vi "Fix Saturated Sin.vi"(9 "start index (0)":i32, 11 "Waveform":dbl[](array[numeric])) -> (0 "RMS value":dbl format="%0.2p", 1 "Rising":i32, 2 "1/2 Period":i32, 3 "Falling":i32, 4 "Sat. Ind":u64, 5 "Peak Amplitude":dbl, 6 "Error":dbl format="%0.6f", 7 "Waveform Graph":dbl[][](graph))   [LabVIEW 2017]
uses:
  <vilib>/Analysis/baseanly.llb/Mean (DBL).vi
  <vilib>/measure/madcrms.llb/Basic Averaged DC-RMS for 1 Chan.vi
  <vilib>/measure/NI_MAPro.lvlib
  <vilib>/Analysis/NI_AALPro.lvlib
  <vilib>/Analysis/2dsp.llb/Real FFT.vi
  <vilib>/measure/mamon.llb/Trigger Detection for 1 Channel.vi
  Crabtree-Lab-Panel--master/Crabtree LAB Panel/Lab Panel V2/program files/Global 1.vi
  <vilib>/Analysis/NI_AALBase.lvlib
panel:
  out "Waveform Graph 3":dbl[](graph)
  out "x-y":dbl[](array[numeric])
  out "Waveform Graph 2":dbl[][](graph)
  in  "O/P Sin Scaler":dbl=1.0
  in  "Threshoild level":dbl=5.0 format="%#_13g"
  in  "Scaling":dbl=1.0
  # "e"
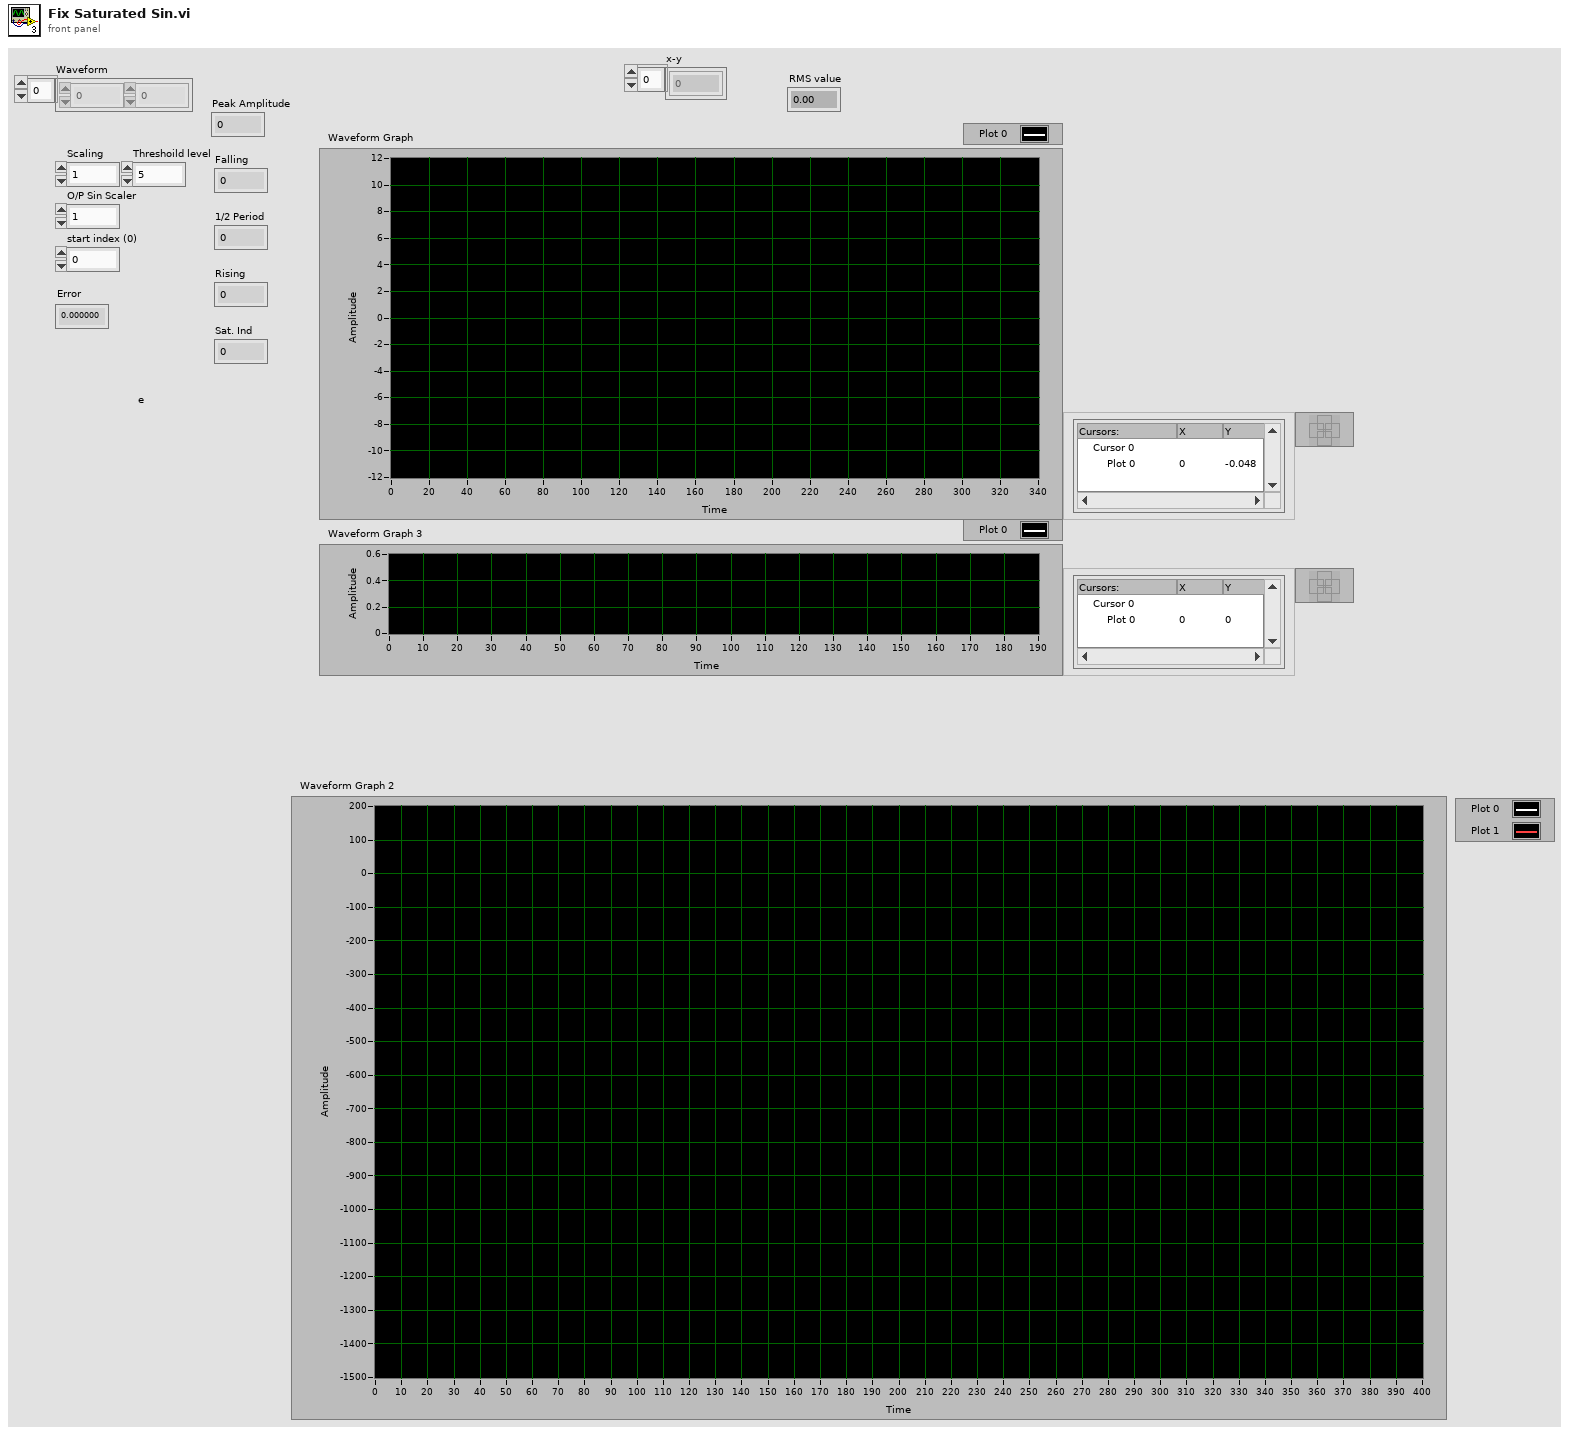
[diagram p1: front panel]
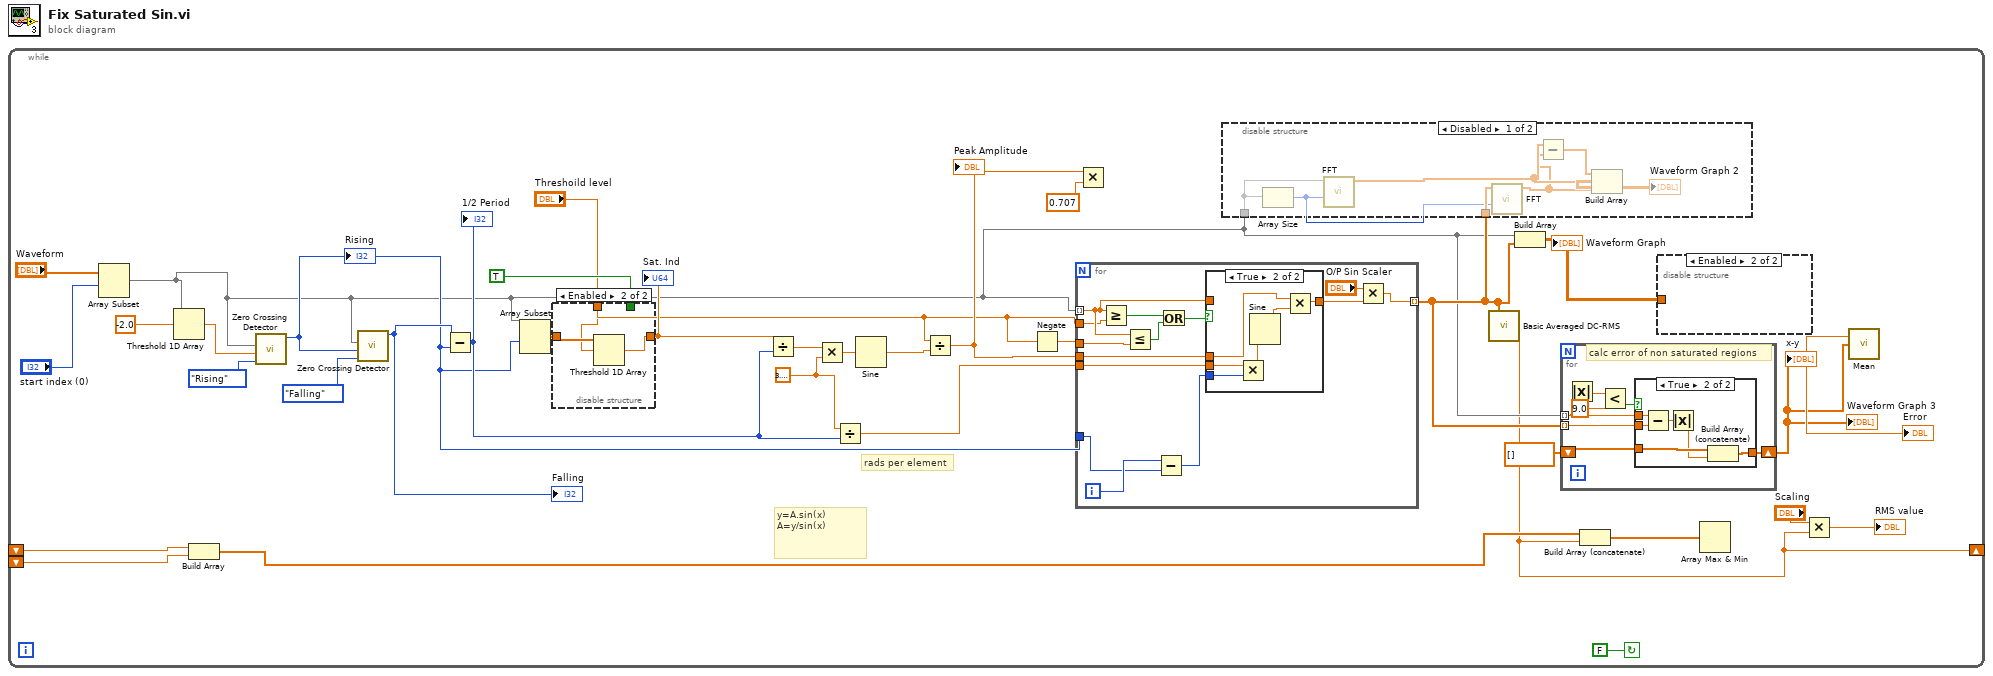
[diagram p0: block diagram]
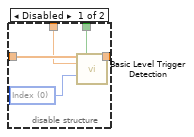
[diagram p3: hidden frame]
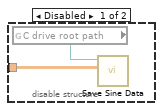
[diagram p4: hidden frame]
diagram:
  n1 = while {
    shift-right: [w2] -> _
    shift-left: _ -> [w16]
    shift-left: _ -> [w17]
    stop <- FALSE continue-if-true
    w25 = 3.141592653589793
    # "y=A.sin(x)\nA=y/sin(x)"
    # "rads per element"
    n2 = Array Subset(array="Waveform", index="start index (0)") -> (w6:dbl[])  [unwired: 1 in]
    n3 = Threshold 1D Array(2:-2.0 ("threshold y"), 3:w6) -> (0:w11:dbl)  [unwired: 1 in]
    n4 = Build Array(w17, w16) -> (w15:dbl[])
    n5 = call "Zero Crossing Detector.vi"("Direction"=enum16{"Rising", "Falling"}."Rising", "offset"=w11, "Y"=w6) -> ("X"=w22:i32)  [unwired: 8 in]
    "Rising" <- w22
    n6 = call "Zero Crossing Detector.vi"("Direction"=enum16{"Rising", "Falling"}."Falling", "offset"=w22, "Y"=w6) -> ("X"=w29:i32)  [unwired: 8 in]
    "Falling" <- w29
    n7 = Subtract(x=w29, y=w22) -> (x-y=w24:i32)
    "1/2 Period" <- w24
    n8 = Array Subset(array=w6, index=w22) -> (w31:dbl[])  [unwired: 1 in]
    n9 = disable-structure shown="Enabled" {
      disable-tunnel: [w54 w55] -> w32
      disable-tunnel: w31 -> [w53 w57]
      disable-tunnel: TRUE ("reset") -> [w51 _]
      disable-tunnel: "Threshoild level" -> [w50 w56]
      frame Disabled {
        w52 = u16 0 items=["Index", "Time"] ("location mode")
        n10 = call-poly <vilib>:"Basic Level Trigger Detection.vi"("signal in"=w53, "reset"=w51, "level"=w50, "location mode"=w52) -> ("trigger location"=w54:dbl)  [unwired: 9 in, 2 out]
      }
      frame Enabled {
        n11 = Threshold 1D Array(2:w56, 3:w57) -> (0:w55:dbl)  [unwired: 1 in]
      }
    }
    "Sat. Ind" <- w32
    n12 = Divide(x=w32, y=w24) -> (x/y=w33:dbl)
    n13 = Multiply(x=w33, y=w25) -> (x*y=w34:dbl)
    n14 = Divide(x=w25, y=w24) -> (x/y=w23:dbl)
    n15 = Sine(x=w34) -> (sin(x)=w35:dbl)
    n16 = Divide(x="Threshoild level", y=w35) -> (x/y=w21:dbl)
    "Peak Amplitude" <- w21
    n17 = Negate(x="Threshoild level") -> (-x=w19:dbl)
    n18 = for {
      tunnel: w6 -> [w73] mode=indexing
      tunnel: "Threshoild level" -> [w72]
      tunnel: w23 -> [w80]
      tunnel: w21 -> [w79]
      tunnel: [w68] -> w10 mode=indexing
      tunnel: w22 -> [w77]
      tunnel: w19 -> [w70]
      i -> [w78]
      n19 = Greater Or Equal?(x=w73, y=w72) -> (x >= y?=w74:bool)
      n20 = Less Or Equal?(x=w73, y=w70) -> (x <= y?=w71:bool)
      n21 = Subtract(x=w78, y=w77) -> (x-y=w76:i32)
      n22 = Or(x=w74, y=w71) -> (x .or. y?=w75:bool)
      n23 = case shown="True" w75 {
        tunnel: [w81 w82] -> w69
        tunnel: w73 -> [w81 _]
        tunnel: w76 -> [_ w87]
        tunnel: w80 -> [_ w86]
        tunnel: w79 -> [_ w83]
        frame False {
        }
        frame True {
          n24 = Multiply(x=w86, y=w87) -> (x*y=w85:dbl)
          n25 = Sine(x=w85) -> (sin(x)=w84:dbl)
          n26 = Multiply(x=w83, y=w84) -> (x*y=w82:dbl)
        }
      }
      n27 = Multiply(x="O/P Sin Scaler", y=w69) -> (x*y=w68:dbl)
    }
    n28 = Multiply(x=w21, y=0.707) -> ()  [unwired: 1 out]
    n29 = disable-structure shown="Disabled" {
      disable-tunnel: w6 -> [w66 _]
      disable-tunnel: w10 -> [w65 _]
      frame Disabled {
        n30 = Array Size(array=w66) -> (size(s)=w64:i32)
        n31 = call-poly <vilib>:"FFT.vi"("FFT size"=w64, "X"=w66) -> ("FFT {X}"=w62:cdb[])  [unwired: 8 in, 1 out]
        n32 = call-poly <vilib>:"FFT.vi"("FFT size"=w64, "X"=w65) -> ("FFT {X}"=w61:cdb[])  [unwired: 8 in, 1 out]
        n33 = Subtract(x=w62, y=w61) -> (x-y=w60:cdb[])
        n34 = Build Array(w60, w62, w61) -> (→"Waveform Graph 2":cdb[][])
      }
      frame Enabled {
      }
    }
    n35 = call-poly <vilib>:"Basic Averaged DC-RMS.vi"("signal in"=w10) -> ("RMS value"=w2:dbl)  [unwired: 7 in, 3 out]
    n36 = Build Array(w6, w10) -> (w13:dbl[][])
    "Waveform Graph" <- w13
    n37 = for {
      tunnel: w10 -> [w42] mode=indexing
      tunnel: w6 -> [w41] mode=indexing
      shift-right: [w36] -> w4
      shift-left: dbl[] [] -> [w37]
      # "calc error of non saturated regions"
      n38 = Absolute Value(x=w41) -> (abs(x)=w40:dbl)
      n39 = Less?(x=w40, y=9.0) -> (x < y?=w38:bool)
      n40 = case shown="True" w38 {
        tunnel: w42 -> [_ w49]
        tunnel: w41 -> [_ w48]
        tunnel: w37 -> [w43 w47]
        tunnel: [w43 w45] -> w36
        frame False {
        }
        frame True {
          n41 = Subtract(x=w48, y=w49) -> (x-y=w46:dbl)
          n42 = Absolute Value(x=w46) -> (abs(x)=w44:dbl)
          n43 = Build Array (concatenate)(w47, w44) -> (w45:dbl[])
        }
      }
    }
    "x-y" <- w4
    "Waveform Graph 3" <- w4
    n44 = Build Array (concatenate)(w15, w2) -> (w14:dbl[])
    n45 = disable-structure shown="Enabled" {
      disable-tunnel: w13 -> [w59 _]
      frame Disabled {
        n46 = global read "Global 1.vi" "C drive root path"() -> (w58:path)
        n47 = call "Save Sine Data.vi"("2D data"=w59, "Path"=w58) -> ()  [unwired: 10 in]
      }
      frame Enabled {
      }
    }
    n48 = Array Max & Min(array=w14) -> ()  [unwired: 4 out]
    n49 = Multiply(x="Scaling", y=w2) -> (x*y=→"RMS value":dbl)
    n50 = call-poly <vilib>:"Mean.vi"("X"=w4) -> ("mean"=→"Error":dbl)  [unwired: 1 out]
  }
